vi "PNG&GIF.vi"() -> ()   [LabVIEW 2013]
panel:
  out "new picture":picture
  in  "PNG path":path
  in  "GIF path":path
  in  "AniGIF":refnum<k7>(container)
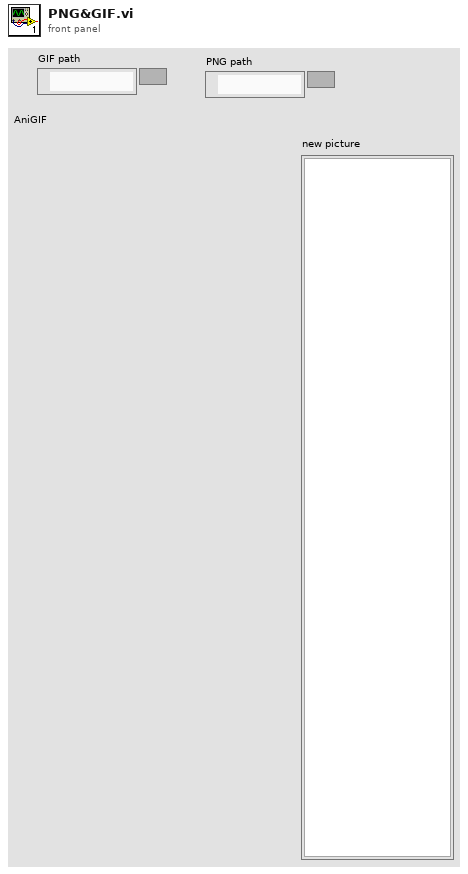
[diagram p1: front panel]
types:
  T1 = typedef "imagedata.ctl" = cluster{"image type":i32, "image depth":i32, "image":u8[], "mask":u8[], "colors":u32[], "Rectangle":cluster{"left":i16, "top":i16, "right":i16, "bottom":i16}}
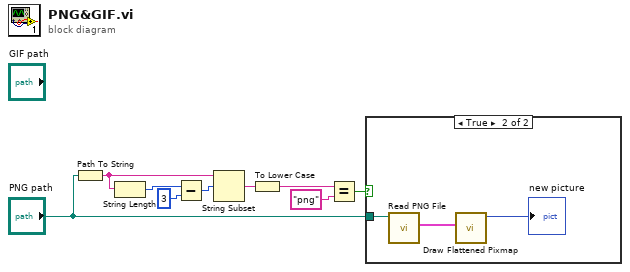
[diagram p0: block diagram]
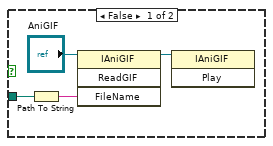
[diagram p2: hidden frame]
diagram:
  n1 = Path To String(path="PNG path") -> (string=w8:string)
  n2 = String Length(string=w8) -> (length=w7:i32)
  n3 = Subtract(x=w7, y=3) -> (x-y=w6:i32)
  n4 = String Subset(string=w8, offset (0)=w6) -> (substring=w4:string)  [unwired: 1 in]
  n5 = To Lower Case(string=w4) -> (all lower case string=w3:string)
  n6 = Equal?(x=w3, y="png") -> (x = y?=w1:bool)
  n7 = case shown="True" w1 {
    tunnel: "PNG path" -> [w11 w16]
    frame False {
      n8 = Path To String(path=w11) -> (string=w10:string)
      n9 = invoke class="IAniGIF" method="ReadGIF"(reference="AniGIF", "FileName"=w10) -> (reference out=w13:refnum<k7>)  [unwired: 2 in, 3 out]
      n10 = invoke class="IAniGIF" method="Play"(reference=w13) -> ()  [unwired: 2 in, 3 out]
    }
    frame True {
      n11 = call <vilib>:"Read PNG File.vi"("path to PNG file"=w16) -> ("image data"=w15:T1)  [unwired: 8 in, 2 out]
      n12 = call <vilib>:"Draw Flattened Pixmap.vi"("image data"=w15) -> ("new picture"=→"new picture":picture)  [unwired: 8 in]
    }
  }
